vi "Write LabVIEW version.vi"(8 "error in (no error)":errorcluster, 10 "LabVIEW version":string, 11 "LV DEV in":refnum<class "LV DEV.lvclass">) -> (0 "error out":errorcluster, 3 "LV DEV out":refnum<class "LV DEV.lvclass">)   [LabVIEW 2016, in "LV DEV.lvclass"]
uses:
  LV DEV.lvclass
  LV DEV.lvclass/LV DEV.ctl
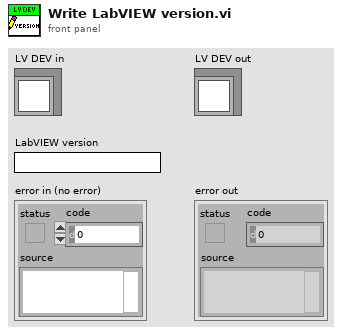
[diagram p1: front panel]
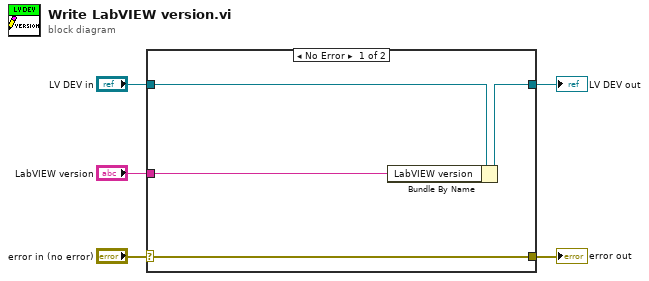
[diagram p0: block diagram]
diagram:
  n1 = case shown="No Error" "error in (no error)" {
    selector: "error in (no error)" -> [w9 w10]
    tunnel: [w9 w10] -> w4
    tunnel: [w7 w11] -> w2
    tunnel: "LV DEV in" -> [w8 w11]
    tunnel: "LabVIEW version" -> [w6 _]
    frame No Error {
      n2 = Bundle By Name(cluster=w8, "LabVIEW version"=w6) -> (w7:refnum<class "LV DEV.lvclass">)
    }
    frame Error {
    }
  }
  "error out" <- w4
  "LV DEV out" <- w2
